vi "Control Init.vi"(7 "VolatusAPI":refnum<class "VolatusAPI.lvclass">, 8 "error in (no error)":errorcluster, 10 "JSON":string, 11 "2WayValve in":refnum<class "2WayValve.lvclass">) -> (0 "error out":errorcluster, 3 "2WayValve out":refnum<class "2WayValve.lvclass">)   [LabVIEW 2020, in "VolatusGUI.lvlib" / "2WayValve.lvclass"]
uses:
  2WayValve.lvclass
  2WayValve.lvclass/2WayValve.ctl
  Volatus/VolatusAPI/VolatusAPI.lvclass
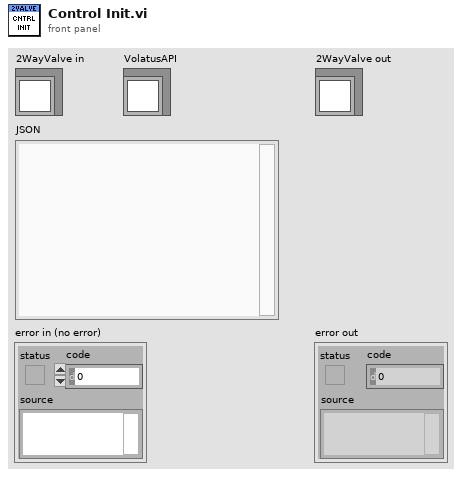
[diagram p1: front panel]
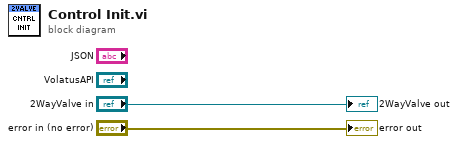
[diagram p0: block diagram]
diagram:
  "error out" <- "error in (no error)"
  "2WayValve out" <- "2WayValve in"
